vi "act-0026-02-cor.vi"() -> ()   [LabVIEW 2010]
uses:
  lv_02/lv_02.lvlib
panel:
  out "f(tc)":dbl[](array[numeric])
  out "Graphe f(tc)":cluster{"Y":dbl[], "Y":dbl[]}[](graph)
  out "MTTF":dbl
  out "tc":dbl[](array[numeric])
  out "dN(tc)":u32[](array[numeric])
  out "tdeb":dbl[](array[numeric])
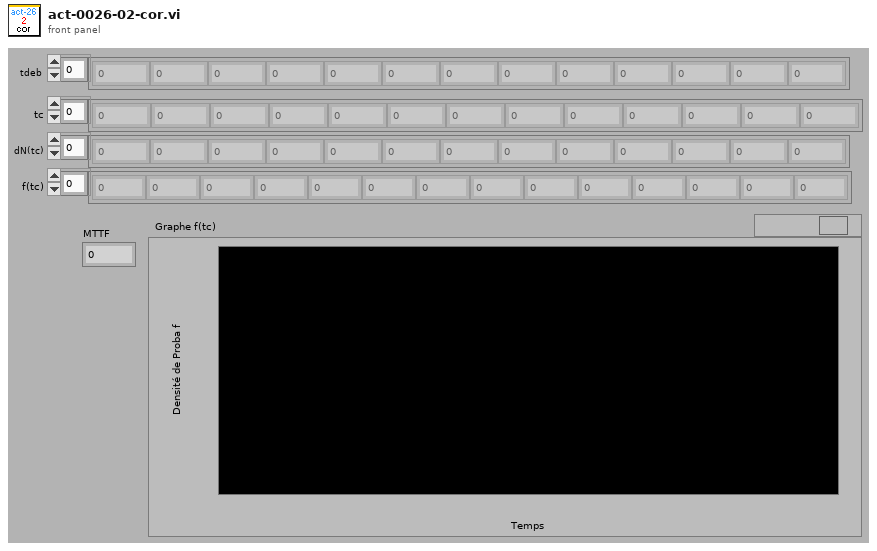
[diagram p1: front panel]
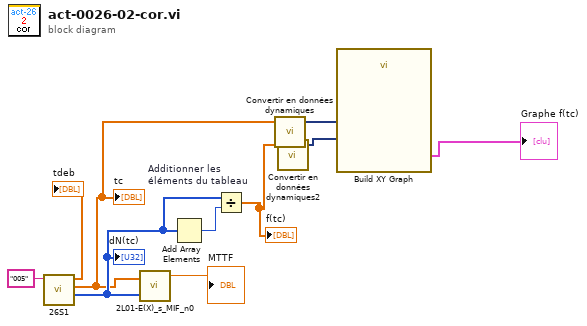
[diagram p0: block diagram]
diagram:
  n1 = call "26S1.vi"("src"="005") -> ("dN(tc)"=w5:u32[], "tc"=w4:dbl[], "tdeb"=→"tdeb":dbl[])  [unwired: 6 in, 2 out]
  "dN(tc)" <- w5
  "tc" <- w4
  n2 = call "2L01-E(X)_s_MIF_n0.vi"("ni"=w5, "xic"=w4) -> ("E(X)"=→"MTTF":dbl)  [unwired: 2 out]
  n3 = Add Array Elements "Additionner les éléments du tableau"(numeric array=w5) -> (sum=w6:u32)
  n4 = Divide(x=w5, y=w6) -> (x/y=w2:dbl[])
  "f(tc)" <- w2
  n5 = call "Convertir en données dynamiques"("Array"=w4) -> ("Dynamic Data Type"=w3:dynamicdata)  [unwired: 3 in]
  n6 = call "Convertir en données dynamiques2"("Array"=w2) -> ("Dynamic Data Type"=w1:dynamicdata)  [unwired: 3 in]
  n7 = call "Build XY Graph"("Y Input"=w1, "X Input"=w3) -> ("XY Graph"=→"Graphe f(tc)":cluster{"Y":dbl[], "Y":dbl[]}[])  [unwired: 3 in, 6 out]
